vi "REQ Acquire Humidity.vi"(8 "error in":errorcluster, 10 "Acquire Humidity":bool) -> (0 "error out":errorcluster)   [LabVIEW 2016, in "Environment Chamber.lvlib"]
doc: "_____\nCreated using DQMH Event Scripter 6.1.0.128."
uses:
  Environment Chamber.lvlib
  REQ Acquire Humidity Argument--cluster.ctl
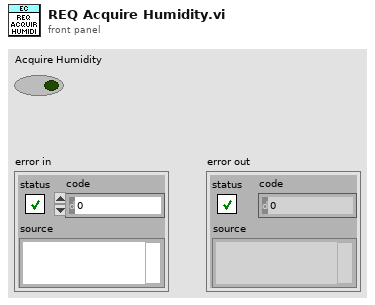
[diagram p1: front panel]
types:
  T1 = typedef "Environment Chamber.lvlib/REQ Acquire Humidity Argument--cluster.ctl" = cluster{"Acquire Humidity":bool}
  T2 = typedef "Environment Chamber.lvlib/Request Events--cluster.ctl" = cluster{"Stop Module":refnum<user-event>, "Show Panel":refnum<user-event>, "Hide Panel":refnum<user-event>, "Get Module Execution Status":refnum<user-event>, "Show Diagram":refnum<user-event>, "REQ Initialize Hardware":refnum<user-event>, "REQ Configure Parameter":refnum<user-event>, "REQ Acquire Data":refnum<user-event>, "REQ Acquire Humidity":refnum<user-event>, "REQ Close Ref":refnum<user-event>, "Broad Humidity Data":refnum<user-event>, "REQ Wakeup_helper_loop":refnum<user-event>, "REQ Retry EC":refnum<user-event>}
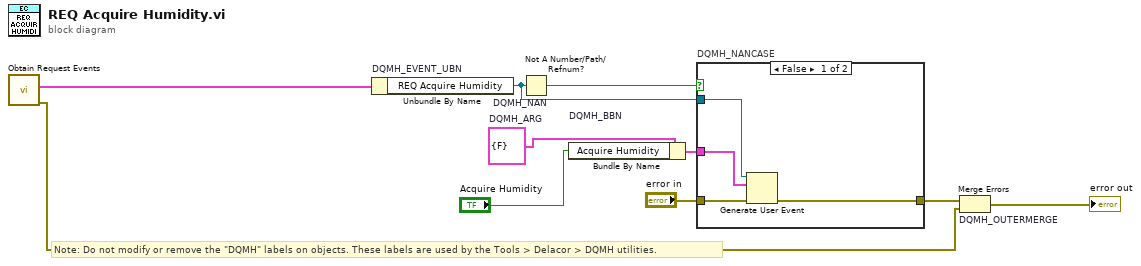
[diagram p0: block diagram]
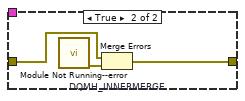
[diagram p2: hidden frame]
diagram:
  w4 = T1 {"Acquire Humidity"=FALSE}  # DQMH_ARG
  # "Note: Do not modify or remove the \"DQMH\" labels on objects. These labels are used by the Tools > Delacor > DQMH utilities."
  n1 = call "Obtain Request Events.vi"() -> ("error out"=w2:errorcluster, "Environment Chamber Request Events"=w1:T2)  [unwired: 10 in]
  n2 = Unbundle By Name "DQMH_EVENT_UBN"(w1) -> ("REQ Acquire Humidity"=w6:refnum<user-event>)
  n3 = Not A Number/Path/Refnum? "DQMH_NAN"(number/path/refnum=w6) -> (NaN/Path/Refnum?=w7:bool)
  n4 = Bundle By Name "DQMH_BBN"(cluster=w4, "Acquire Humidity"="Acquire Humidity") -> (w8:T1)
  n5 = case "DQMH_NANCASE" shown="False" w7 {
    tunnel: "error in" -> [w14 w17]
    tunnel: [w13 w16] -> w5
    tunnel: w6 -> [w12 _]
    tunnel: w8 -> [w11 _]
    frame False {
      n6 = Generate User Event(user event=w12, event data cluster=w11, error in=w14) -> (error out=w13:errorcluster)  [unwired: 1 in, 1 out]
    }
    frame True {
      n7 = call "Module Not Running--error.vi"() -> ("error out"=w15:errorcluster)  [unwired: 11 in]
      n8 = Merge Errors "DQMH_INNERMERGE"(w17, w15) -> (w16:errorcluster)
    }
  }
  n9 = Merge Errors "DQMH_OUTERMERGE"(w5, w2) -> (→"error out":errorcluster)
